vi "triangle_source.vi"(2 "protect_scan":bool, 3 "pause":bool, 4 "triangle_control":T1 {"end_source / V" format="%#_13g"; "lower_volt_limit / V" format="%#_13g"; "upper_volt_limit / V" format="%#_13g"; "step_voltage / V" format="%#_13g"; "init_source / V" format="%#_13g"}) -> (0 "terminate?":bool, 1 "output_signal / V":dbl format="%#_13g")   [LabVIEW 2014]
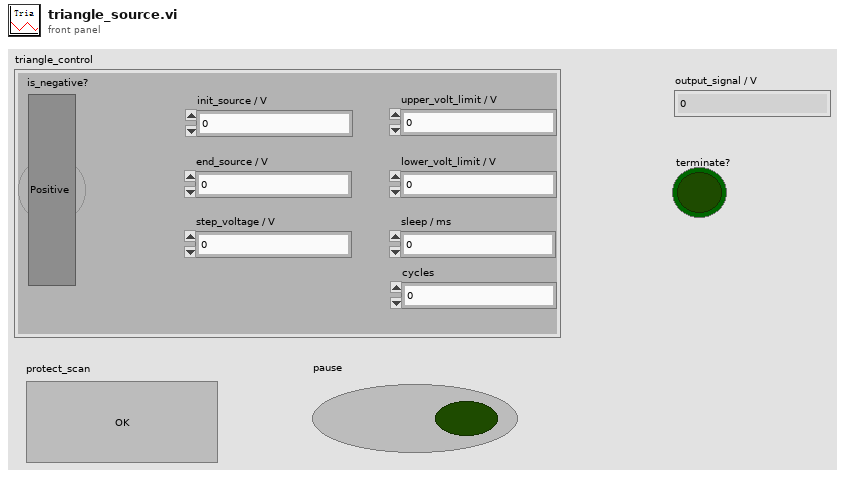
[diagram p1: front panel]
types:
  T1 = cluster{"init_source / V":dbl, "step_voltage / V":dbl, "upper_volt_limit / V":dbl, "lower_volt_limit / V":dbl, "sleep / ms":u32, "is_negative?":bool, "cycles":u32, "end_source / V":dbl}
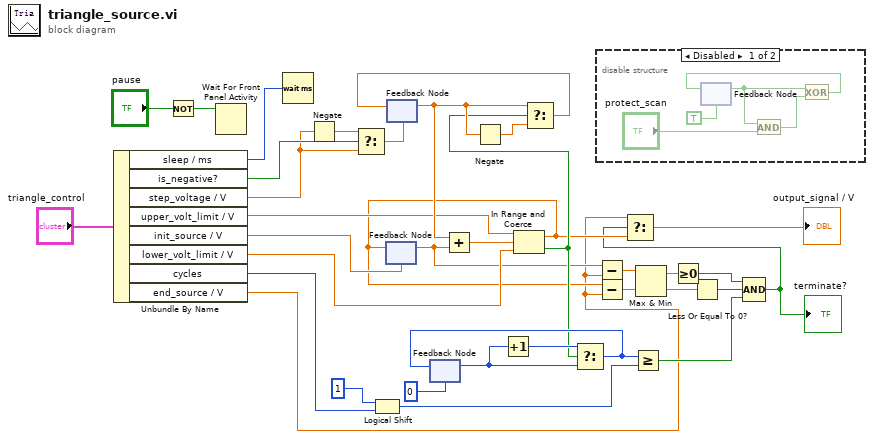
[diagram p0: block diagram]
diagram:
  n1 = Unbundle By Name("triangle_control") -> ("sleep / ms"=w29:u32, "is_negative?"=w28:bool, "step_voltage / V"=w27:dbl, "upper_volt_limit / V"=w26:dbl, "init_source / V"=w25:dbl, "lower_volt_limit / V"=w24:dbl, "cycles"=w20:u32, "end_source / V"=w2:dbl)
  n2 = Not(x="pause") -> (.not. x?=w3:bool)
  n3 = Wait For Front Panel Activity(3:w3) -> ()  [unwired: 2 in, 1 out]
  n4 = Wait (ms)(milliseconds to wait=w29) -> ()  [unwired: 1 out]
  n5 = Negate(x=w27) -> (-x=w34:dbl)
  n6 = Select(t=w34, s=w28, f=w27) -> (s? t:f=w35:dbl)
  n7 = Logical Shift(y=i16 1, x=w20) -> (x << y=w18:u32)
  n8 = feedback #1(w25) -> (w14:dbl)
  n9 = feedback #2(w35) -> (w33:dbl)
  n10 = feedback #3(0) -> (w22:i32)
  n11 = Add(x=w33, y=w14) -> (x+y=w15:dbl)
  n12 = Negate(x=w33) -> (-x=w32:dbl)
  n13 = Increment(x=w22) -> (x+1=w21:i32)
  n14 = In Range and Coerce(upper limit=w26, x=w15, lower limit=w24) -> (coerced(x)=w5:dbl, In Range?=w16:bool)
  n15 = feedback-in #1(w5) -> ()
  n16 = Select(t=w33, s=w16, f=w32) -> (s? t:f=w31:dbl)
  n17 = feedback-in #2(w31) -> ()
  n18 = Select(t=w21, s=w16, f=w22) -> (s? t:f=w17:i32)
  n19 = feedback-in #3(w17) -> ()
  n20 = disable-structure shown="Disabled" {
    frame Disabled {
      n21 = feedback #4(TRUE) -> (w38:bool)
      n22 = And(x=w38, y="protect_scan") -> (x .and. y?=w36:bool)
      n23 = Exclusive Or(1:w36, 2:w38) -> (0:w37:bool)
      n24 = feedback-in #4(w37) -> ()
    }
    frame Enabled {
    }
  }
  n25 = Subtract(x=w14, y=w2) -> (x-y=w13:dbl)
  n26 = Subtract(x=w5, y=w2) -> (x-y=w12:dbl)
  n27 = Greater Or Equal?(x=w17, y=w18) -> (x >= y?=w7:bool)
  n28 = Max & Min(x=w13, y=w12) -> (max(x,y)=w11:dbl, min(x,y)=w10:dbl)
  n29 = Greater Or Equal To 0?(x=w11) -> (x >= 0?=w9:bool)
  n30 = Less Or Equal To 0?(x=w10) -> (x <= 0?=w8:bool)
  n31 = Compound Arithmetic op=AND(w9, w8, w7) -> (w1:bool)
  "terminate?" <- w1
  n32 = Select(t=w2, s=w1, f=w5) -> (s? t:f=→"output_signal / V":dbl)
